vi "CTRE_Phoenix_CANdle_Animate.vi"   [LabVIEW 2020]
doc: "Lights up the LEDs in the chosen animation pattern."
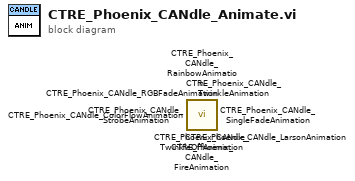
[diagram p0: block diagram]
diagram:
  n1 = call <vilib>:"CTRE_Phoenix_CANdle_TwinkleOffAnimation.vi"() -> ()  [unwired: 14 in, 2 out]
  n2 = call <vilib>:"CTRE_Phoenix_CANdle_TwinkleAnimation.vi"() -> ()  [unwired: 14 in, 2 out]
  n3 = call <vilib>:"CTRE_Phoenix_CANdle_StrobeAnimation.vi"() -> ()  [unwired: 14 in, 2 out]
  n4 = call <vilib>:"CTRE_Phoenix_CANdle_SingleFadeAnimation.vi"() -> ()  [unwired: 14 in, 2 out]
  n5 = call <vilib>:"CTRE_Phoenix_CANdle_RGBFadeAnimation.vi"() -> ()  [unwired: 14 in, 2 out]
  n6 = call <vilib>:"CTRE_Phoenix_CANdle_RainbowAnimation.vi"() -> ()  [unwired: 14 in, 2 out]
  n7 = call <vilib>:"CTRE_Phoenix_CANdle_LarsonAnimation.vi"() -> ()  [unwired: 14 in, 2 out]
  n8 = call <vilib>:"CTRE_Phoenix_CANdle_FireAnimation.vi"() -> ()  [unwired: 14 in, 2 out]
  n9 = call <vilib>:"CTRE_Phoenix_CANdle_ColorFlowAnimation.vi"() -> ()  [unwired: 14 in, 2 out]
